vi "PNDT - assemble version info.vi"(7 "other info":string, 8 "#bytes [2]":i32=2, 9 "start index":i32, 10 "version label":string, 11 "version bytes":u8[](array[numeric])) -> (2 "version info":string)   [LabVIEW 2026, in "MicroPulse_Driver.lvlib"]
uses:
  MicroPulse_Driver.lvlib
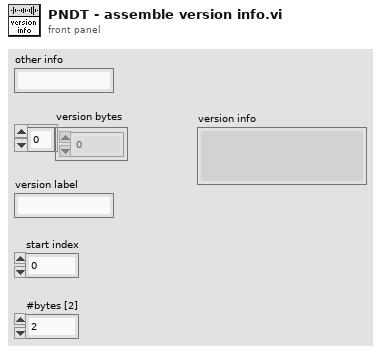
[diagram p1: front panel]
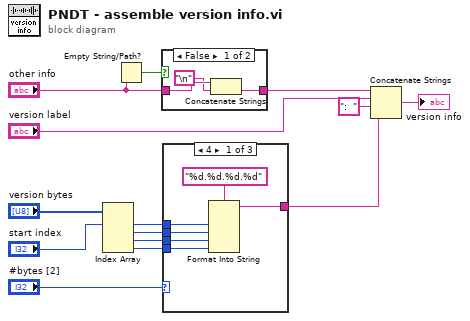
[diagram p0: block diagram]
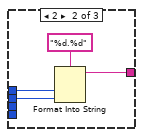
[diagram p3: hidden frame]
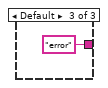
[diagram p4: hidden frame]
diagram:
  n1 = Index Array(array="version bytes", index #1="start index") -> (element #1=w13:u8, element #2=w12:u8, element #3=w11:u8, element #4=w10:u8)  [unwired: 3 in]
  n2 = Empty String/Path?(string/path="other info") -> (empty?=w5:bool)
  n3 = case shown="False" w5 {
    tunnel: "other info" -> [w17 _]
    tunnel: [w16 _] -> w6
    frame False {
      n4 = Concatenate Strings(w17, "\n") -> (w16:string)
    }
    frame True {
    }
  }
  n5 = case shown="4" "#bytes [2]" {
    tunnel: w13 -> [w23 w27 _]
    tunnel: w12 -> [w22 w26 _]
    tunnel: w11 -> [w21 _ _]
    tunnel: w10 -> [w20 _ _]
    tunnel: [w18 w24 "error"] -> w3
    frame 4 {
      n6 = Format Into String(format string="%d.%d.%d.%d", w23, w22, w21, w20) -> (resulting string=w18:string)  [unwired: 2 in, 1 out]
    }
    frame 2 {
      n7 = Format Into String(format string="%d.%d", w27, w26) -> (resulting string=w24:string)  [unwired: 2 in, 1 out]
    }
    frame Default {
    }
  }
  n8 = Concatenate Strings(w6, "version label", ":  " ("string"), w3) -> (→"version info":string)
